vi "ptr_write2ptr_read.vi"(1 "ptr_write":u32) -> (0 "ptr_read":u32)   [LabVIEW 2013]
uses:
  GlobleVar/segment_size.vi
  GlobleVar/stack_size.vi
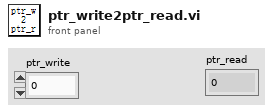
[diagram p1: front panel]
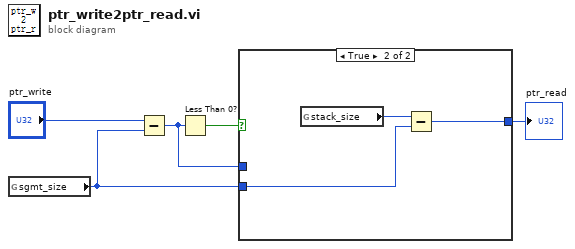
[diagram p0: block diagram]
diagram:
  n1 = global read "segment_size.vi" "sgmt_size"() -> (w1:i32)
  n2 = Subtract(x="ptr_write", y=w1) -> (x-y=w2:u32)
  n3 = Less Than 0?(x=w2) -> (x < 0?=w4:bool)
  n4 = case shown="True" w4 {
    tunnel: [w6 w7] -> w3
    tunnel: w2 -> [w6 _]
    tunnel: w1 -> [_ w8]
    frame False {
    }
    frame True {
      n5 = global read "stack_size.vi" "stack_size"() -> (w9:i32)
      n6 = Subtract(x=w9, y=w8) -> (x-y=w7:i32)
    }
  }
  "ptr_read" <- w3
